vi "Control Panel.vi"(8 "error in (no error)":errorcluster, 11 "Stepper in":refnum<class "Stepper.lvclass">) -> (0 "error out":errorcluster, 3 "Stepper out":refnum<class "Stepper.lvclass">)   [LabVIEW 2009, in "Stepper.lvclass"]
uses:
  Stepper.lvclass
panel:
  in  "Desired Wavelength":dbl[unit] step=1e-09
  out "Current Wavelength":dbl[unit] step=1e-09
  in  "endprgm":bool
  in  "Start/Stop":bool
  in  "Speed":dbl[unit]=5e-09
  out "Direction":bool
  out "Coil Status":bool[](array[boolean])=[TRUE, TRUE, TRUE, TRUE, TRUE, TRUE, TRUE, TRUE]
  # "Ti-Sapph Wavelength Control"
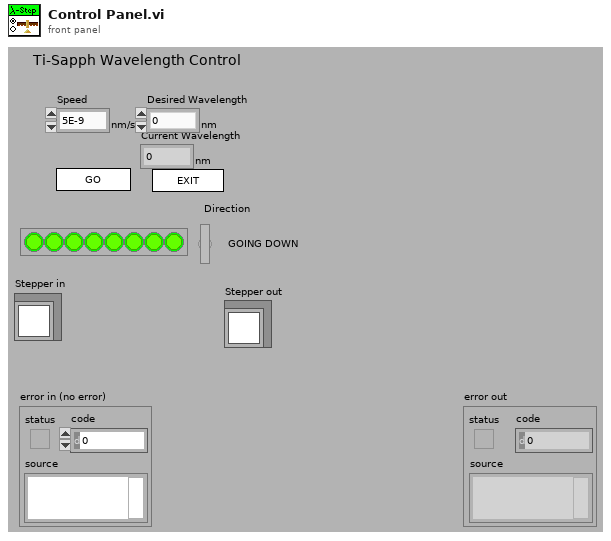
[diagram p1: front panel]
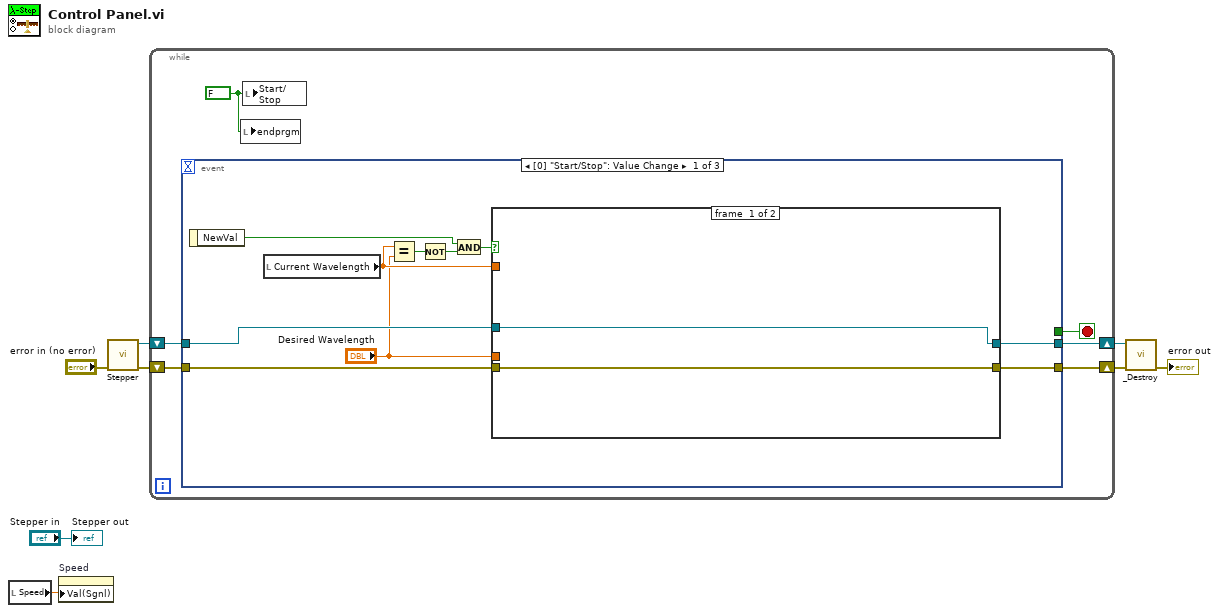
[diagram p0: block diagram]
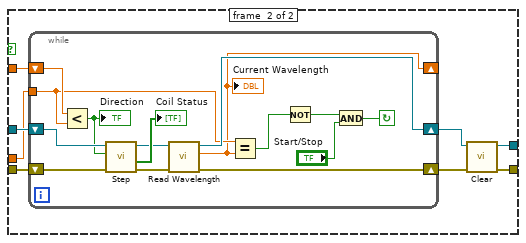
[diagram p2: hidden frame]
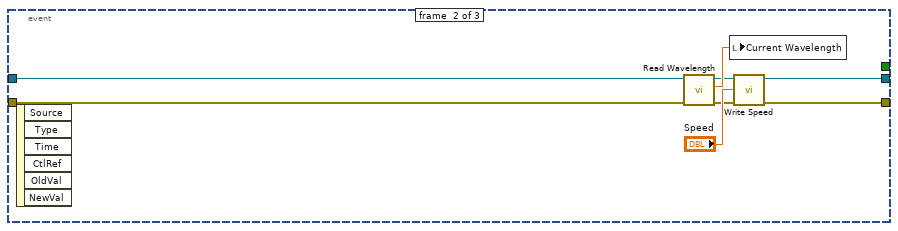
[diagram p3: hidden frame]
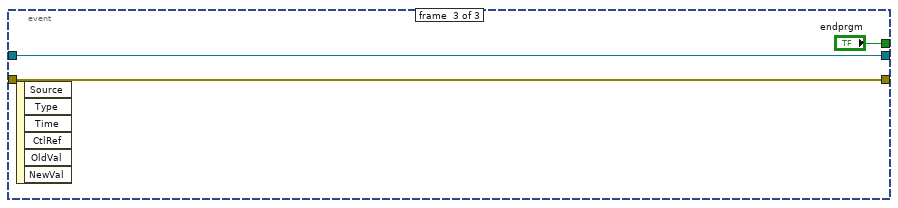
[diagram p4: hidden frame]
diagram:
  n1 = local read "Speed"() -> (w1:dbl[unit])
  n2 = property on="Speed" class="DigNum (strict)"("Val(Sgnl)"=w1) -> ()  [unwired: 2 in, 2 out]
  n3 = call "Stepper.vi"("error in (no error)"="error in (no error)") -> ("error out"=w5:errorcluster, "Stepper out"=w4:refnum<class "Stepper.lvclass">)  [unwired: 9 out]
  n4 = while {
    shift-right: [w12] -> w6
    shift-left: w4 -> [w9]
    shift-right: [w10] -> w3
    shift-left: w5 -> [w11]
    stop <- w14 stop-if-true
    w13 = FALSE
    n5 = event shown="[0] \"Start/Stop\": Value Change" {
      selector: _ -> [_ _ _]
      dyn-events: _ -> [_ _ _]
      timeout: _ -> [_ _ _]
      tunnel: [_ _ "endprgm"] -> w14
      tunnel: [w24 w56 w59] -> w12
      tunnel: w9 -> [w23 w53 w59]
      tunnel: w11 -> [w22 w51 w58]
      tunnel: [w21 w55 w58] -> w10
      event #0 {
        n6 = event-data() -> ("NewVal"=w19:bool)  [unwired: 1 out]
        n7 = local read "Current Wavelength"() -> (w16:dbl[unit])
        n8 = Equal?(x=w16, y="Desired Wavelength") -> (x = y?=w20:bool)
        n9 = Not(x=w20) -> (.not. x?=w17:bool)
        n10 = And(x=w19, y=w17) -> (x .and. y?=w18:bool)
        n11 = case shown="True" w18 {
          tunnel: [w26 w29] -> w24
          tunnel: w23 -> [w26 w33]
          tunnel: w22 -> [w25 w32]
          tunnel: [w25 w27] -> w21
          tunnel: "Desired Wavelength" -> [_ w31]
          tunnel: w16 -> [_ w30]
          frame #0 {
          }
          frame #1 {
            n12 = while {
              shift-right: [w45] -> w34
              shift-left: w33 -> [w48]
              shift-right: [w43] -> w28
              shift-left: w32 -> [w47]
              shift-right: [w35] -> _
              shift-left: w30 -> [w37]
              tunnel: w31 -> [w36]
              stop <- w40 continue-if-true
              n13 = Less?(x=w37, y=w36) -> (x < y?=w42:bool)
              "Direction" <- w42
              n14 = call "Step.vi"("error in"=w47, "Up?"=w42, "Stepper.lvclass"=w48) -> ("error out"=w44:errorcluster, "Coil Status"=→"Coil Status":bool[], "Stepper.lvclass out"=w46:refnum<class "Stepper.lvclass">)  [unwired: 6 out]
              n15 = call-dynamic "Read Wavelength.vi"("error in (no error)"=w44, "Stepper.lvclass in"=w46) -> ("error out"=w43:errorcluster, "Current Wavelength"=w35:dbl[unit], "Stepper.lvclass out"=w45:refnum<class "Stepper.lvclass">)  [unwired: 7 out]
              "Current Wavelength" <- w35
              n16 = Equal?(x=w36, y=w35) -> (x = y?=w39:bool)
              n17 = Not(x=w39) -> (.not. x?=w38:bool)
              n18 = And(x=w38, y="Start/Stop") -> (x .and. y?=w40:bool)
            }
            n19 = call-dynamic "Clear.vi"("error in (no error)"=w28, "Stepper in"=w34) -> ("error out"=w27:errorcluster, "Stepper out"=w29:refnum<class "Stepper.lvclass">)  [unwired: 8 out]
          }
        }
      }
      event #1 {
        n20 = event-data() -> ()  [unwired: 7 out]
        n21 = call-dynamic "Read Wavelength.vi"("error in (no error)"=w51, "Stepper.lvclass in"=w53) -> ("error out"=w50:errorcluster, "Current Wavelength"=w54:dbl[unit], "Stepper.lvclass out"=w52:refnum<class "Stepper.lvclass">)  [unwired: 7 out]
        n22 = local write "Current Wavelength"(w54) -> ()
        n23 = call-dynamic "Write Speed.vi"("error in (no error)"=w50, "Speed"="Speed", "Stepper.lvclass in"=w52) -> ("error out"=w55:errorcluster, "Stepper.lvclass out"=w56:refnum<class "Stepper.lvclass">)  [unwired: 7 out]
      }
      event #2 {
        n24 = event-data() -> ()  [unwired: 7 out]
      }
    }
    n25 = local write "endprgm"(w13) -> ()
    n26 = local write "Start/Stop"(w13) -> ()
  }
  n27 = call-dynamic "_Destroy.vi"("error in (no error)"=w3, "Stepper in"=w6) -> ("error out"=→"error out":errorcluster)  [unwired: 9 out]
  "Stepper out" <- "Stepper in"
